vi "20170516-lecture4-2 prof StateMachine.vi"() -> ()   [LabVIEW 2014]
panel:
  out "Logined":bool
  in  "stop":bool
  out "array":bool[](array[boolean])
  in  "Button":T1
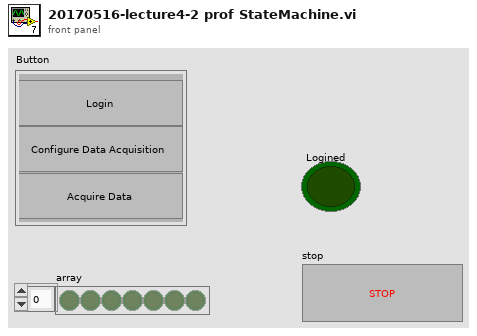
[diagram p1: front panel]
types:
  T1 = cluster{"OK Button":bool, "OK Button 2":bool, "OK Button 3":bool}
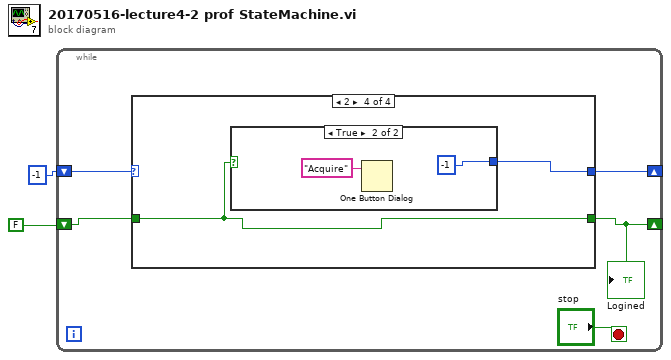
[diagram p0: block diagram]
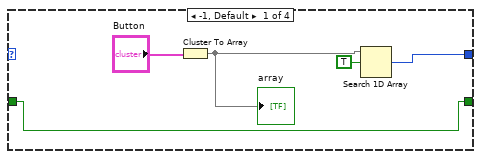
[diagram p2: hidden frame]
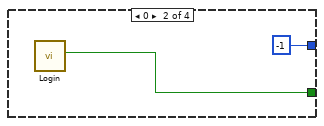
[diagram p3: hidden frame]
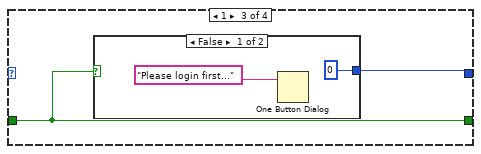
[diagram p4: hidden frame]
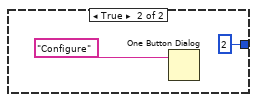
[diagram p5: hidden frame]
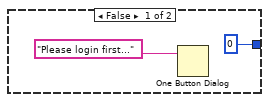
[diagram p6: hidden frame]
diagram:
  n1 = while {
    shift-right: [w5] -> _
    shift-left: -1 -> [w6]
    shift-right: [w4] -> _
    shift-left: FALSE -> [w3]
    stop <- "stop" stop-if-true
    n2 = case shown="2" w6 {
      tunnel: [w9 -1 w15 w21] -> w5
      tunnel: [w8 w13 w16 w22] -> w4
      tunnel: w3 -> [w8 _ w16 w22]
      frame -1, Default {
        n3 = Cluster To Array(cluster="Button") -> (array=w11:bool[])
        "array" <- w11
        n4 = Search 1D Array(1D array=w11, element=TRUE) -> (index of element=w9:i32)  [unwired: 1 in]
      }
      frame 0 {
        n5 = call "Login.vi"() -> ("Correct"=w13:bool)  [unwired: 11 in]
      }
      frame 1 {
        n6 = case shown="False" w16 {
          tunnel: [0 2] -> w15
          frame False {
            n7 = One Button Dialog(message="Please login first...") -> ()  [unwired: 1 in, 1 out]
          }
          frame True {
            n8 = One Button Dialog(message="Configure") -> ()  [unwired: 1 in, 1 out]
          }
        }
      }
      frame 2 {
        n9 = case shown="True" w22 {
          tunnel: [0 -1 ("index of element")] -> w21
          frame False {
            n10 = One Button Dialog(message="Please login first...") -> ()  [unwired: 1 in, 1 out]
          }
          frame True {
            n11 = One Button Dialog(message="Acquire") -> ()  [unwired: 1 in, 1 out]
          }
        }
      }
    }
    "Logined" <- w4
  }
